vi "Launcher Template (Top Level VI).vi"() -> ()   [LabVIEW 2021, in "Architecture.lvlib"]
uses:
  Architecture.lvlib
  Typedefs/FGV Ref. Modules Function.ctl
  Typedefs/Enum_Module_Name.ctl
  Error_Log/LogRotate/LogRotate.lvclass
  Typedefs/Module References.ctl
  Typedefs/Message.ctl
  SubVIs/Module Template SM.vi
panel:
  out "error out":errorcluster
  in  "Loading Bar":u8(slide) caption="Loading Database..." max=100 step=1 scale=0.0..100.0
  # "APPLICATION LAUNCHER"
  # "Juan Pérez Rodríguez"
  # "https://CtrlVIStudios.com"
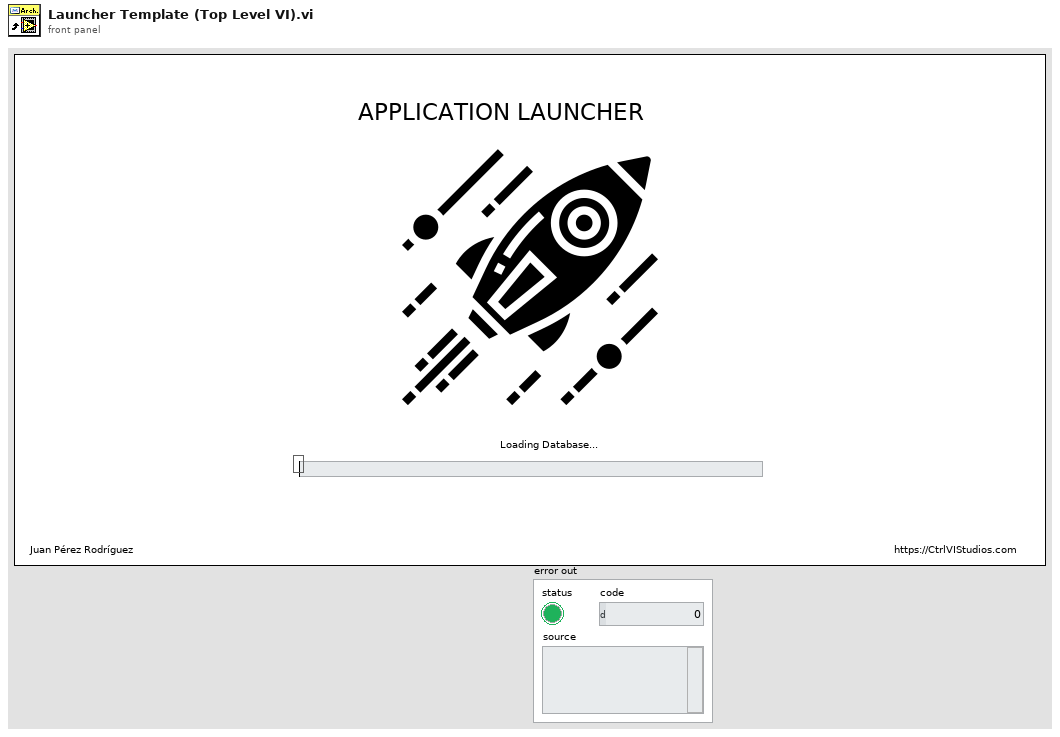
[diagram p1: front panel]
types:
  T1 = typedef "Architecture.lvlib/Enum_Module_Name.ctl" = enum16{"Configuration", "Error_Handler", "Log", "Database", "Controller"}
  T2 = cluster{"ModuleName":T1, "ShowFP":bool, "StatesTracking Enabled":bool}[]
  T3 = typedef "Architecture.lvlib/FGV Ref. Modules Function.ctl" = enum16{"Init ", "Add Module", "Get Module", "Get All", "Add Asynchronous Run Ref", "Dispose"}
  T4 = typedef "Architecture.lvlib/Module References.ctl" = cluster{"ModuleName":T1, "Queue":refnum<queue>, "user event":refnum<user-event>, "VI Refnum":refnum<vi>, "ShowFP":bool, "StatesTracking Enabled":bool}
  T5 = enum32{"invalid app kind", "Development System", "Run Time System", "Student Edition", "Embedded LabVIEW", "Evaluation", "Custom"}
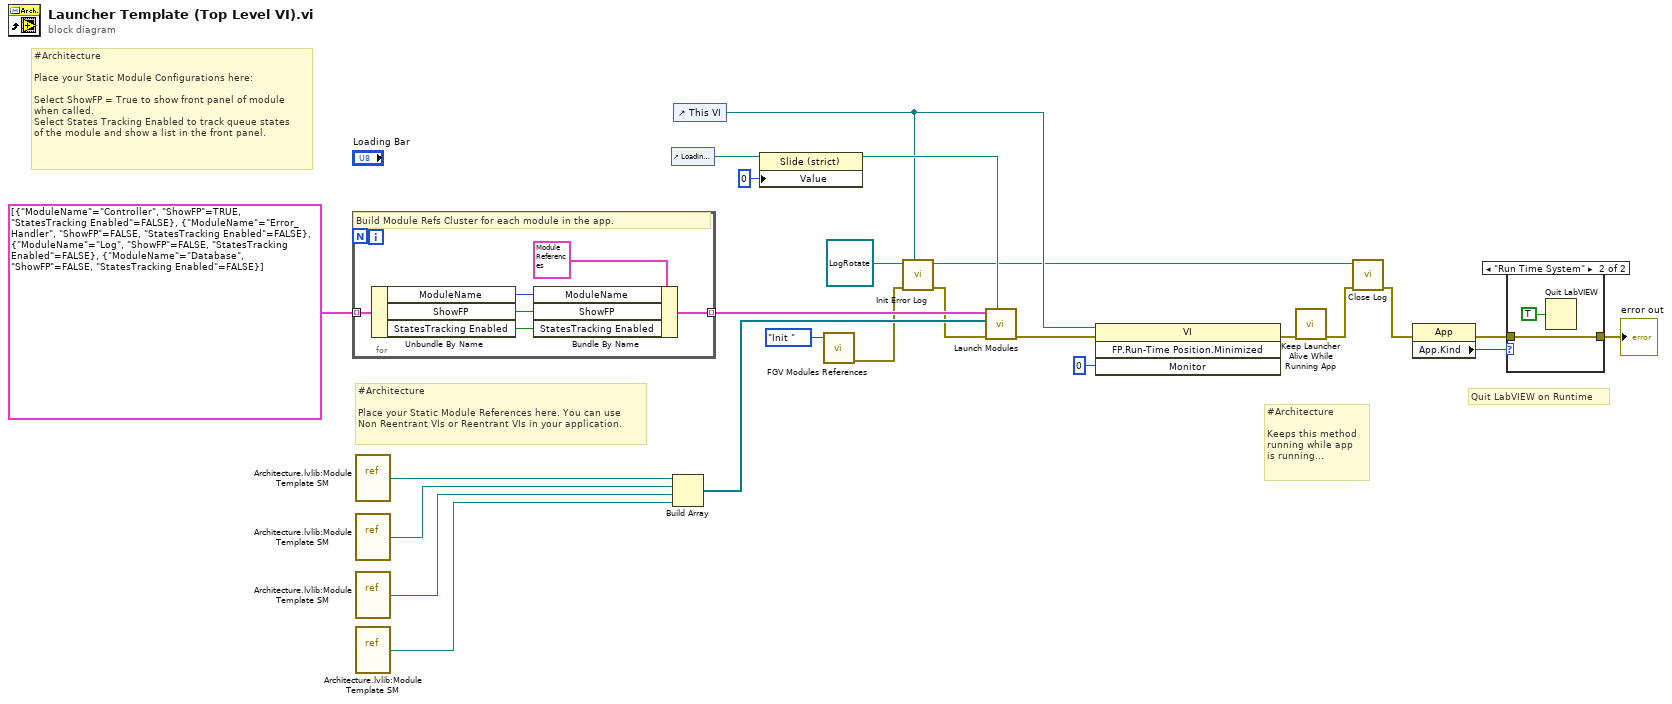
[diagram p0: block diagram]
diagram:
  # "#Architecture\n\nKeeps this method \nrunning while app \nis running..."
  # "Quit LabVIEW on Runtime"
  # "#Architecture\n\nPlace your Static Module References here. You can use\nNon Reentrant VIs or Reentrant VIs in your application."
  # "#Architecture\n\nPlace your Static Module Configurations here:\n\nSelect ShowFP = True to show front panel of module\nwhen called. \nSelect States Tracking Enabled to track queue states\nof the module and show a list in the front panel."
  n1 = for {
    tunnel: T2 [{"ModuleName"=enum."Controller", "ShowFP"=TRUE, "StatesTracking Enabled"=FALSE}, {"ModuleName"=enum."Error_Handler", "ShowFP"=FALSE, "StatesTracking Enabled"=FALSE}, {"ModuleName"=enum."Log", "ShowFP"=FALSE, "StatesTracking Enabled"=FALSE}, {"ModuleName"=enum."Database", "ShowFP"=FALSE, "StatesTracking Enabled"=FALSE}] -> [w29] mode=indexing
    tunnel: [w25] -> w23 mode=indexing
    # "Build Module Refs Cluster for each module in the app."
    n2 = Unbundle By Name(w29) -> ("ModuleName"=w28:T1, "ShowFP"=w27:bool, "StatesTracking Enabled"=w26:bool)
    n3 = Bundle By Name(cluster=T4 {"ModuleName"=enum."Controller", "Queue"=refnum, "user event"=refnum, "VI Refnum"=refnum, "ShowFP"=FALSE, "StatesTracking Enabled"=FALSE} ("Module_Refs"), "ModuleName"=w28, "ShowFP"=w27, "StatesTracking Enabled"=w26) -> (w25:T4)
  }
  n4 = vi-ref "Architecture.lvlib:Module Template SM.vi"() -> (w14:refnum<vi>)
  n5 = vi-ref "Architecture.lvlib:Module Template SM.vi"() -> (w13:refnum<vi>)
  n6 = vi-ref "Architecture.lvlib:Module Template SM.vi"() -> (w12:refnum<vi>)
  n7 = vi-ref "Architecture.lvlib:Module Template SM.vi"() -> (w11:refnum<vi>)
  n8 = control-ref of="Loading Bar"() -> (w22:refnum<vi>)
  n9 = Build Array(w14, w13, w12, w11) -> (w17:refnum<vi>[])
  n10 = control-ref of="This VI"() -> (w5:refnum<vi>)
  n11 = property class="Slide (strict)"(reference=w22, "Value"=u8 0) -> (reference out=w20:refnum<vi>)  [unwired: 1 in, 1 out]
  n12 = call "FGV Modules References.vi"("FGV Ref. Function In"=FGV_Ref._Modules_Function."Init ") -> ("error out"=w7:errorcluster)  [unwired: 8 in, 2 out]
  n13 = call "Init Error Log.vi"("TopLevel"=w5, "error in (no error)"=w7, "LogRotate in"=refnum<class "LogRotate.lvclass"> refnum) -> ("error out"=w6:errorcluster, "LogRotate out"=w3:refnum<class "LogRotate.lvclass">)  [unwired: 7 in]
  n14 = call "Launch Modules.vi"("Loading Bar Ref In"=w20, "error in (no error)"=w6, "App Modules Refs"=w17, "Modules Info In"=w23) -> ("error out"=w18:errorcluster)  [unwired: 7 in]
  n15 = invoke class="VI" method="FP.Run-Time Position.Minimized"(reference=w5, error in=w18, "Monitor"=i16 0) -> (error out=w16:errorcluster)  [unwired: 1 in, 3 out]
  n16 = call "Keep Launcher Alive While Running App.vi"("error in (no error)"=w16) -> ("error out"=w2:errorcluster)  [unwired: 10 in]
  n17 = call "Close Log.vi"("error in (no error)"=w2, "LogRotate in"=w3) -> ("error out"=w1:errorcluster)  [unwired: 8 in, 1 out]
  n18 = property class="App"(error in=w1) -> (error out=w10:errorcluster, "App.Kind"=w8:T5)  [unwired: 1 in, 1 out]
  n19 = case shown="\"Run Time System\"" w8 {
    tunnel: w10 -> [w31 w33]
    tunnel: [w31 w33] -> w9
    frame Default {
    }
    frame "Run Time System" {
      n20 = Quit LabVIEW(quit? (T)=TRUE) -> ()
    }
  }
  "error out" <- w9
